vi "Get image date.vi"(8 "error in (no error)":errorcluster, 11 "Simulated_CCD_Camera in":refnum<class "Simulated_CCD_Camera.lvclass">) -> (0 "error out":errorcluster, 3 "Simulated_CCD_Camera out":refnum<class "Simulated_CCD_Camera.lvclass">)   [LabVIEW 2018, in "Simulated_CCD_Camera.lvclass"]
doc: "Get the time stamp (in UTC) at star of exposure"
uses:
  Simulated_CCD_Camera.lvclass
  Simulated_CCD_Camera.lvclass/Simulated_CCD_Camera.ctl
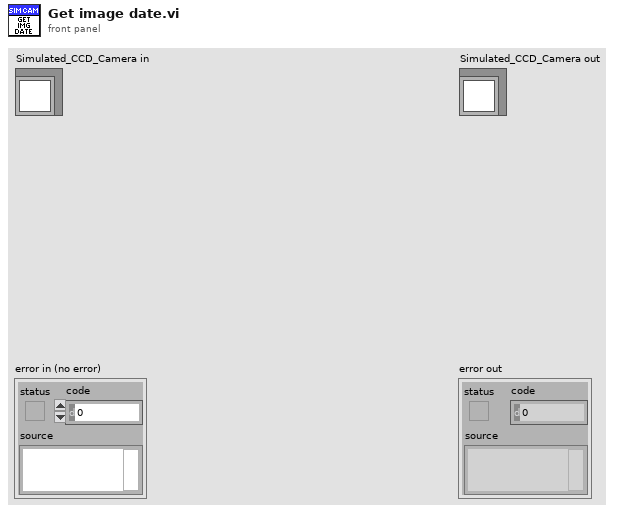
[diagram p1: front panel]
types:
  T1 = typedef "LVDateTimeRec.ctl" = cluster{"fractional second":dbl, "second":i32, "minute":i32, "hour":i32, "day of month":i32, "month":i32, "year":i32, "day of week":i32, "day of year":i32, "DST":i32}
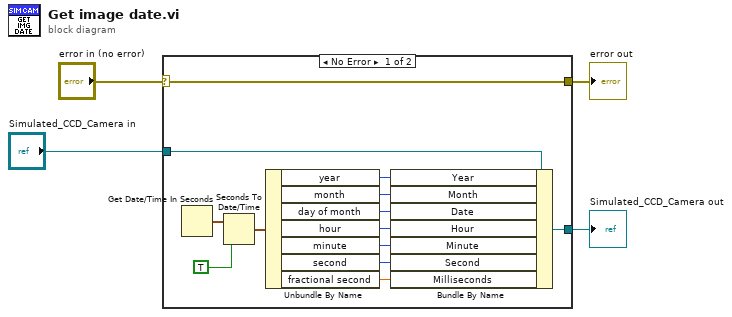
[diagram p0: block diagram]
diagram:
  n1 = case shown="No Error" "error in (no error)" {
    selector: "error in (no error)" -> [w17 w19]
    tunnel: [w17 w19] -> w3
    tunnel: [w6 w18] -> w1
    tunnel: "Simulated_CCD_Camera in" -> [w7 w18]
    frame No Error {
      n2 = Get Date/Time In Seconds() -> (seconds since 1Jan1904=w16:timestamp)
      n3 = Seconds To Date/Time(time stamp (now)=w16, to UTC (F)=TRUE) -> (date time rec=w15:T1)
      n4 = Unbundle By Name(w15) -> ("year"=w14:i32, "month"=w13:i32, "day of month"=w12:i32, "hour"=w11:i32, "minute"=w10:i32, "second"=w9:i32, "fractional second"=w8:dbl)
      n5 = Bundle By Name(cluster=w7, "Year"=w14, "Month"=w13, "Date"=w12, "Hour"=w11, "Minute"=w10, "Second"=w9, "Milliseconds"=w8) -> (w6:refnum<class "Simulated_CCD_Camera.lvclass">)
    }
    frame Error {
    }
  }
  "error out" <- w3
  "Simulated_CCD_Camera out" <- w1
